vi "StellarNet Write Operating Parameters to XML.vi"(8 "error in (no error)":errorcluster, 10 "Operating Parameters":T1(array[cluster]) {"Digitizer Clock Rate Setting" min=1 max=3; "Optical Smoothing Level" min=0 max=4 step=1; "Number of Scans to Average" min=1 max=10000 step=1}, 11 "XML File Path":path) -> (0 "error out":errorcluster)   [LabVIEW 2023]
uses:
  StellarNet SpectraWiz-Chemo Globals.vi
  <vilib>/Utility/xml.llb/Write to XML File(string).vi
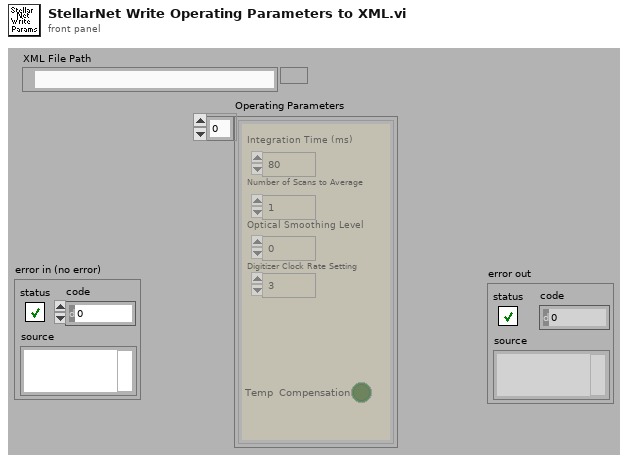
[diagram p1: front panel]
types:
  T1 = cluster{"Integration Time (ms)":i32, "Number of Scans to Average":i32, "Optical Smoothing Level":i32, "Digitizer Clock Rate Setting":i32, "Temp  Compensation ":bool}[]
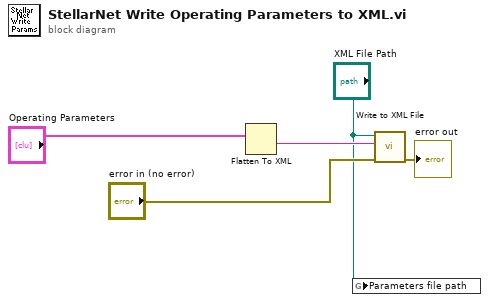
[diagram p0: block diagram]
diagram:
  n1 = Flatten To XML(6:"Operating Parameters") -> (2:w5:string)
  n2 = global write "StellarNet SpectraWiz-Chemo Globals.vi" "Parameters file path"("XML File Path") -> ()
  n3 = call-poly <vilib>:"Write to XML File.vi"("error in (no error)"="error in (no error)", "XML Input"=w5, "XML File Path"="XML File Path") -> ("error out"=→"error out":errorcluster)  [unwired: 6 in, 2 out]
